vi "invert joystick cluster values.vi"(8 "Invert Y":bool, 9 "Invert X":bool, 10 "Slide":cluster{u32, u32}(slide) scale=0.0..7.0, 11 "Joystick Readings":T1) -> (3 "Joystick Readings 2":T1)   [LabVIEW 2012]
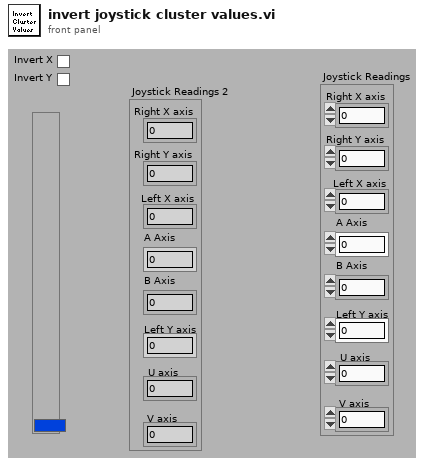
[diagram p1: front panel]
types:
  T1 = cluster{"Right X axis":i32, "Right Y axis":i32, "Left X axis":i32, "A Axis":i32, "B Axis":i32, "Left Y axis":i32, "U axis":i32, "V axis":i32}
  T2 = cluster{"Joystick Readings[0]":i32, "Joystick Readings[1]":i32, "Joystick Readings[2]":i32, "Joystick Readings[3]":i32, "Joystick Readings[4]":i32, "Joystick Readings[5]":i32, "Joystick Readings[6]":i32, "Joystick Readings[7]":i32, "Joystick Readings[8]":i32}
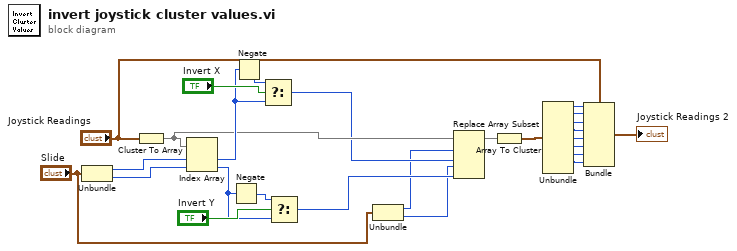
[diagram p0: block diagram]
diagram:
  n1 = Unbundle("Slide") -> (w26:u32, w25:u32)
  n2 = Cluster To Array(cluster="Joystick Readings") -> (array=w18:i32[])
  n3 = Index Array(array=w18, index #1=w26, index #2=w25) -> (element #1=w19:i32, element #2=w21:i32)
  n4 = Negate(x=w21) -> (-x=w22:i32)
  n5 = Negate(x=w19) -> (-x=w20:i32)
  n6 = Select(t=w20, s="Invert X", f=w19) -> (s? t:f=w17:i32)
  n7 = Select(t=w22, s="Invert Y", f=w21) -> (s? t:f=w16:i32)
  n8 = Unbundle("Slide") -> (w14:u32, w13:u32)
  n9 = Replace Array Subset(array=w18, new element #1=w17, index #1=w14, new element #2=w16, index #2=w13) -> (w12:i32[])
  n10 = Array To Cluster(array=w12) -> (cluster=w11:T2)
  n11 = Unbundle(w11) -> ("Joystick Readings[0]"=w9:i32, "Joystick Readings[1]"=w8:i32, "Joystick Readings[2]"=w7:i32, "Joystick Readings[3]"=w6:i32, "Joystick Readings[4]"=w5:i32, "Joystick Readings[5]"=w4:i32, "Joystick Readings[6]"=w3:i32, "Joystick Readings[7]"=w2:i32)  [unwired: 1 out]
  n12 = Bundle(cluster="Joystick Readings", "Right X axis"=w9, "Right Y axis"=w8, "Left X axis"=w7, "A Axis"=w6, "B Axis"=w5, "Left Y axis"=w4, "U axis"=w3, "V axis"=w2) -> (→"Joystick Readings 2":T1)
